vi "Initialize_Comm.vi"(8 "error in (no error)":errorcluster, 10 "Baud rate":T1, 11 "Serial Port in":refnum<visa-resource-name>) -> (0 "error out":errorcluster, 3 "Serial Port out":refnum<visa-resource-name>)   [LabVIEW 2016, in "Chemyx_Syringe_Pump_driver.lvlib"]
doc: "Initializes serial communication using Serial Port in and the selected baud rate.\nBaud rate is an enum. Possible values are 9600 or 38400. Must be set to match setting of the pump."
uses:
  Chemyx_Syringe_Pump_driver.lvlib
  controls/comm_rate_enum.ctl
  <vilib>/Instr/_visa.llb/VISA Configure Serial Port (Instr).vi
panel:
  # "Initializes serial communication using Serial Port in and the selected baud rate.\nBaud rate is an enum. Possible values are 9600 or 38400. Must be set to match setting of the pump."
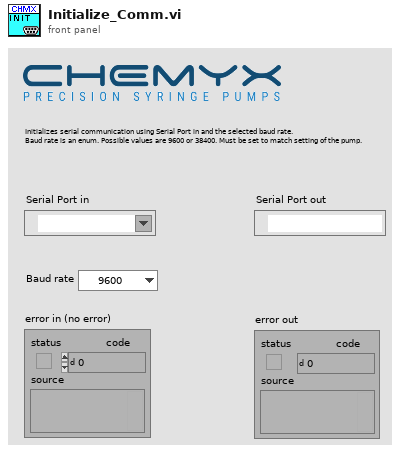
[diagram p1: front panel]
types:
  T1 = typedef "Chemyx_Syringe_Pump_driver.lvlib/comm_rate_enum.ctl" = enum16{"9600", "38400"}
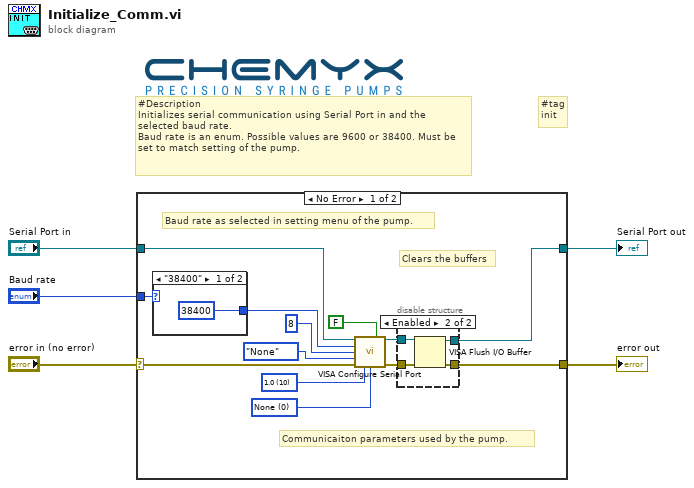
[diagram p0: block diagram]
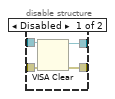
[diagram p2: hidden frame]
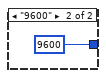
[diagram p3: hidden frame]
diagram:
  # "#tag\ninit"
  # "#Description\nInitializes serial communication using Serial Port in and the selected baud rate.\nBaud rate is an enum. Possible values are 9600 or 38400. Must be set to match setting of the pump."
  n1 = case shown="No Error" "error in (no error)" {
    selector: "error in (no error)" -> [w11 w30]
    tunnel: "Serial Port in" -> [w18 w29]
    tunnel: [w6 w29] -> w4
    tunnel: [w7 w30] -> w2
    tunnel: "Baud rate" -> [w10 _]
    frame No Error {
      w13 = u16 10 items=["1.0"=10, "1.5"=15, "2.0"=20] ("stop bits (10: 1 bit)")
      w14 = u16 0 items=["None", "XON/XOFF", "RTS/CTS", "XON/XOFF & RTS/CTS", "DTR/DSR", "XON/XOFF & DTR/DSR"] ("flow control (0:none)")
      # "Baud rate as selected in setting menu of the pump."
      # "Communicaiton parameters used by the pump."
      # "Clears the buffers"
      n2 = case shown="\"38400\"" w10 {
        tunnel: [u32 38400 ("baud rate (9600)") u32 9600 ("baud rate (9600)")] -> w17
        frame "38400" {
        }
        frame "9600" {
        }
      }
      n3 = call-poly "VISA Configure Serial Port"("VISA resource name"=w18, "Enable Termination\nChar (T)"=FALSE ("Enable Termination\nChar (T)"), "baud rate (9600)"=w17, "data bits (8)"=u16 8, "parity (0:none)"=enum16{"None", "Odd", "Even", "Mark", "Space"}."None", "error in (no error)"=w11, "stop bits (10: 1 bit)"=w13, "flow control (0:none)"=w14) -> ("VISA resource name out"=w8:refnum<visa-resource-name>, "error out"=w9:errorcluster)  [unwired: 6 in]
      n4 = disable-structure shown="Enabled" {
        disable-tunnel: w9 -> [w22 w24]
        disable-tunnel: w8 -> [w21 w26]
        disable-tunnel: [w20 w23] -> w7
        disable-tunnel: [w19 w25] -> w6
        frame Disabled {
          n5 = VISA Clear(VISA resource name=w21, error in (no error)=w22) -> (VISA resource name out=w19:refnum<visa-resource-name>, error out=w20:errorcluster)
        }
        frame Enabled {
          n6 = VISA Flush I/O Buffer(VISA resource name=w26, error in (no error)=w24) -> (VISA resource name out=w25:refnum<visa-resource-name>, error out=w23:errorcluster)  [unwired: 1 in]
        }
      }
    }
    frame Error {
      # "Error in: no initialization"
    }
  }
  "Serial Port out" <- w4
  "error out" <- w2
